vi "Load_Channel_Config_new.vi"(8 "Error in":errorcluster, 11 "configuration file path":path) -> (0 "Error out":errorcluster, 3 "Channel_Information_Control":T1 {"Input Terminal Configuration" items=["default"=-1, "RSE"=10083, "NRSE"=10078, "Differential"=10106, "Pseudodifferential"=12529]})   [LabVIEW 2017]
doc: "Load Channel Information from an XML File"
uses:
  <vilib>/Utility/config.llb/NI_LVConfig.lvlib
  <vilib>/Utility/config.llb/Read Key (String).vi
  typedef/Channel_Information_Control_single.ctl
  typedef/Channel_Information_Control_array.ctl
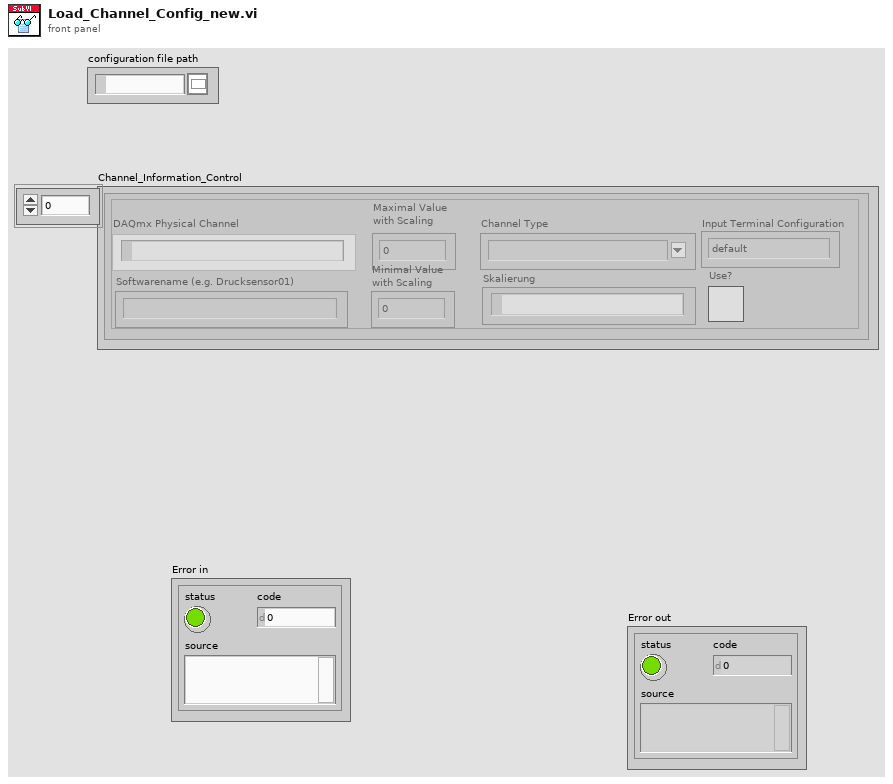
[diagram p1: front panel]
types:
  T1 = typedef "Channel_Information_Control_array.ctl" = T2[]
  T2 = typedef "Channel_Information_Control_single.ctl" = cluster{"DAQmx Physical Channel":tag, "Softwarename (e.g. Drucksensor01)":string, "Maximal Value \nwith Scaling":dbl, "Minimal Value\nwith Scaling":dbl, "Channel Type":string, "Input Terminal Configuration":i32, "Skalierung":tag, "Use?":bool}
  T3 = typedef "NI_LVConfig.lvlib/Config Data RefNum.ctl" = refnum<k1>
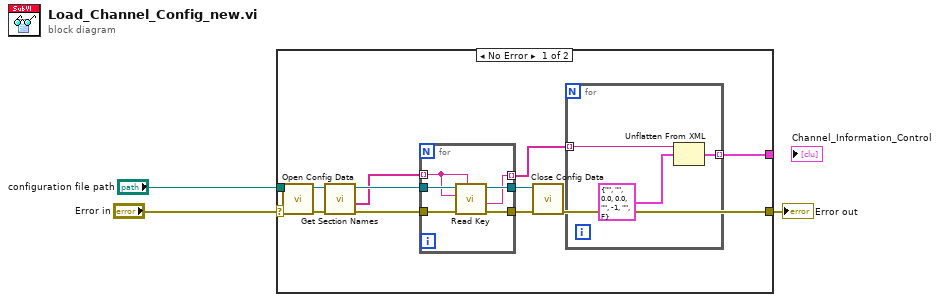
[diagram p0: block diagram]
diagram:
  n1 = case shown="No Error" "Error in" {
    selector: "Error in" -> [w4 w25]
    tunnel: "configuration file path" -> [w15 _]
    tunnel: [w14 w25] -> w2
    tunnel: [w13 _] -> _
    frame No Error {
      n2 = call <vilib>:"Open Config Data.vi"("error in (no error)"=w4, "configuration file path"=w15) -> ("error out"=w8:errorcluster, "refnum"=w9:T3)  [unwired: 7 in, 1 out]
      n3 = call <vilib>:"Get Section Names.vi"("error in (no error)"=w8, "refnum"=w9) -> ("error out"=w10:errorcluster, "section names"=w5:string[], "refnum out"=w6:T3)  [unwired: 7 in]
      n4 = for {
        tunnel: [w24] -> w12
        tunnel: [w23] -> w11
        tunnel: w5 -> [w19] mode=indexing
        tunnel: w10 -> [w22]
        tunnel: [w21] -> w7 mode=indexing
        tunnel: w6 -> [w20]
        n5 = call-poly <vilib>:"Read Key.vi"("section"=w19, "error in (no error)"=w22, "key"=w19, "refnum"=w20) -> ("error out"=w24:errorcluster, "value"=w21:string, "refnum out"=w23:T3)  [unwired: 4 in, 1 out]
      }
      n6 = call <vilib>:"Close Config Data.vi"("error in (no error)"=w12, "refnum"=w11) -> ("error out"=w14:errorcluster)  [unwired: 8 in, 1 out]
      n7 = for {
        tunnel: [w18] -> w13 mode=indexing
        tunnel: w7 -> [w17] mode=indexing
        n8 = Unflatten From XML(xml string=w17, type=T2 {"DAQmx Physical Channel"="", "Softwarename (e.g. Drucksensor01)"="", "Maximal Value \nwith Scaling"=0.0, "Minimal Value\nwith Scaling"=0.0, "Channel Type"="", "Input Terminal Configuration"=-1, "Skalierung"="", "Use?"=FALSE} ("Channel_Information")) -> (value=w18:T2)  [unwired: 1 in, 1 out]
      }
    }
    frame Error {
      # "Don't overwrite Channel Information Control if File Dialog was cancelled"
    }
  }
  "Error out" <- w2
